vi "find or create references.vi"(7 "vi type":T1, 8 "Data Interface VI":string, 9 "Index Cluster Name":string, 10 "Data Cluster Name":string, 11 "LVClassLibrary in":refnum<vi>) -> (0 "error out":errorcluster, 3 "vi refs":T2)   [LabVIEW 2013]
uses:
  Controls/initialized references.ctl
  Controls/interface VI type.ctl
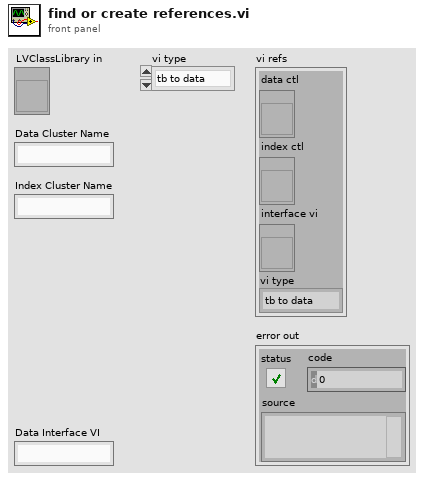
[diagram p1: front panel]
types:
  T1 = typedef "interface VI type.ctl" = enum16{"tb to data", "data to tb"}
  T2 = typedef "initialized references.ctl" = cluster{"data ctl":refnum<vi>, "index ctl":refnum<vi>, "interface vi":refnum<vi>, "vi type":T1}
  T3 = enum32{"invalid VI type", "Standard VI", "Control VI", "Global VI", "Polymorphic VI", "Configuration VI", "SubSystem", "Facade VI", "Method VI"}
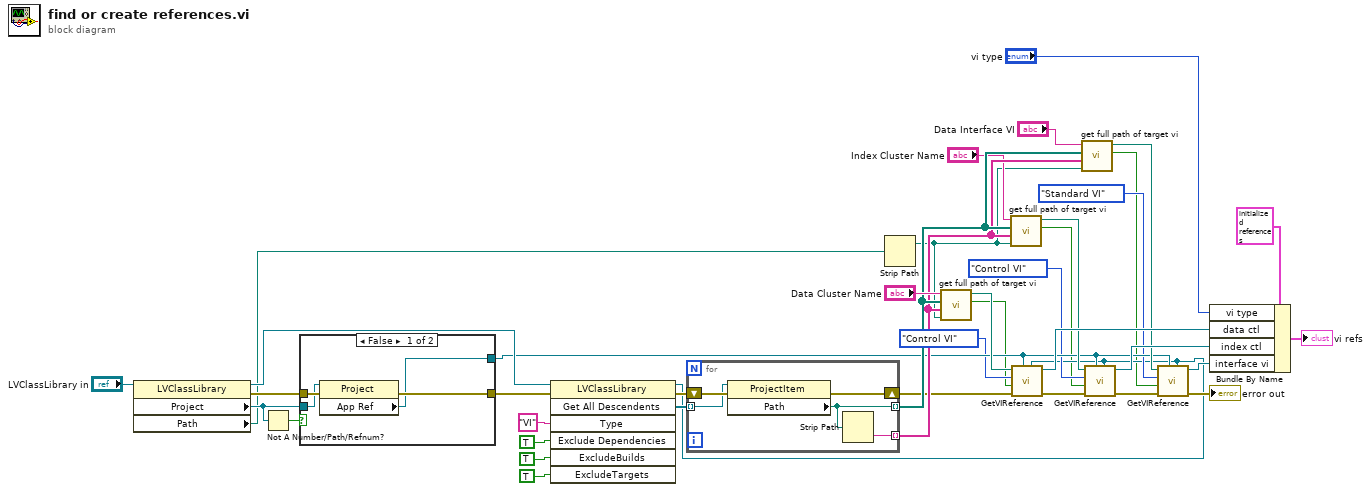
[diagram p0: block diagram]
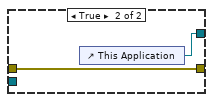
[diagram p2: hidden frame]
diagram:
  n1 = property class="LVClassLibrary"(reference="LVClassLibrary in") -> (reference out=w30:refnum<vi>, error out=w29:errorcluster, "Project"=w27:refnum<vi>, "Path"=w25:path)  [unwired: 1 in]
  n2 = Not A Number/Path/Refnum?(number/path/refnum=w27) -> (NaN/Path/Refnum?=w26:bool)
  n3 = case shown="False" w26 {
    tunnel: w29 -> [w44 w46]
    tunnel: [w43 w46] -> w28
    tunnel: w27 -> [w42 _]
    tunnel: [w41 w45] -> w8
    frame False {
      n4 = property class="Project"(reference=w42, error in=w44) -> (error out=w43:errorcluster, "App Ref"=w41:refnum<vi>)  [unwired: 1 out]
    }
    frame True {
      n5 = control-ref of="This Application"() -> (w45:refnum<vi>)
    }
  }
  n6 = invoke class="LVClassLibrary" method="Get All Descendents"(reference=w30, error in=w28, "Type"="VI", "Exclude Dependencies"=TRUE ("ExcludeDependencies"), "ExcludeBuilds"=TRUE, "ExcludeTargets"=TRUE) -> (reference out=w4:refnum<vi>, error out=w32:errorcluster, "All Descendents"=w31:refnum<vi>[])  [unwired: 1 in, 4 out]
  n7 = for {
    shift-right: [w49] -> w14
    shift-left: w32 -> [w51]
    tunnel: w31 -> [w50] mode=indexing
    tunnel: [w48] -> w22 mode=indexing
    tunnel: [w47] -> w21 mode=indexing
    n8 = property class="ProjectItem"(reference=w50, error in=w51) -> (error out=w49:errorcluster, "Path"=w48:path)  [unwired: 1 out]
    n9 = Strip Path(path=w48) -> (name=w47:string)  [unwired: 1 out]
  }
  n10 = Strip Path(path=w25) -> (stripped path=w18:path)  [unwired: 1 out]
  n11 = call "get full path of target vi.vi"("class folder path"=w18, "class vi names"=w21, "class vi paths"=w22, "vi to qualify"="Data Cluster Name") -> ("not in class"=w3:bool, "full path"=w24:path)  [unwired: 6 in]
  n12 = call "get full path of target vi.vi"("class folder path"=w18, "class vi names"=w21, "class vi paths"=w22, "vi to qualify"="Index Cluster Name") -> ("not in class"=w2:bool, "full path"=w9:path)  [unwired: 6 in]
  n13 = call "GetVIReference.vi"("LVClassLibrary in"=w4, "application reference"=w8, "error in"=w14, "not in class"=w3, "vi type"=T3."Control VI", "file path"=w24) -> ("error out"=w16:errorcluster, "reference out"=w17:refnum<vi>)  [unwired: 4 in]
  n14 = call "get full path of target vi.vi"("class folder path"=w18, "class vi names"=w21, "class vi paths"=w22, "vi to qualify"="Data Interface VI") -> ("not in class"=w1:bool, "full path"=w10:path)  [unwired: 6 in]
  n15 = call "GetVIReference.vi"("LVClassLibrary in"=w4, "application reference"=w8, "error in"=w16, "not in class"=w2, "vi type"=T3."Control VI", "file path"=w9) -> ("error out"=w15:errorcluster, "reference out"=w11:refnum<vi>)  [unwired: 4 in]
  n16 = call "GetVIReference.vi"("LVClassLibrary in"=w4, "application reference"=w8, "error in"=w15, "not in class"=w1, "vi type"=T3."Standard VI", "file path"=w10) -> ("error out"=→"error out":errorcluster, "reference out"=w12:refnum<vi>)  [unwired: 4 in]
  n17 = Bundle By Name(cluster=T2 {"data ctl"=refnum, "index ctl"=refnum, "interface vi"=refnum, "vi type"=enum."tb to data"} ("vi refs"), "vi type"="vi type", "data ctl"=w17, "index ctl"=w11, "interface vi"=w12) -> (→"vi refs":T2)
